vi "APD_filter.vi"(4 "error in":errorcluster, 5 "source of ticks":tag="/Dev1/100MHzTimebase", 6 "counter_filter":tag="Dev1/ctr1", 7 "APD signal":tag="/Dev1/PFI8") -> (0 "error out":errorcluster, 3 "filtered APD":refnum<k21>)   [LabVIEW 2018]
uses:
  <vilib>/DAQmx/create/channels.llb/DAQmx Create Channel (CO-Pulse Generation-Ticks).vi
  <vilib>/DAQmx/configure/trigger.llb/DAQmx Start Trigger (Digital Edge).vi
  <resource>/objmgr/daqmx.rc
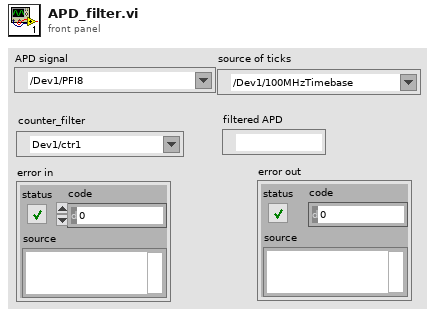
[diagram p1: front panel]
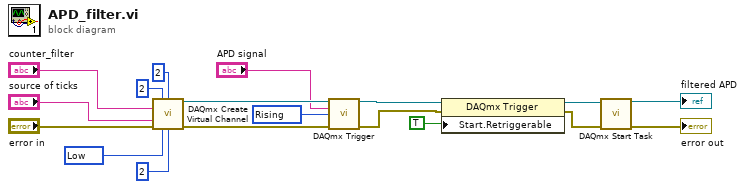
[diagram p0: block diagram]
diagram:
  w8 = 10280 items=["Rising"=10280, "Falling"=10171] ("edge")
  w6 = 10214 items=["High"=10192, "Low"=10214] ("idle state")
  n1 = call-poly <vilib>:"DAQmx Create Virtual Channel.vi"("high ticks"=u32 2, "low ticks"=u32 2, "counter"="counter_filter", "source of ticks"="source of ticks", "error in"="error in", "idle state"=w6, "initial delay"=u32 2) -> ("task out"=w12:refnum<k21>, "error out"=w15:errorcluster)  [unwired: 7 in]
  n2 = call-poly <vilib>:"DAQmx Trigger.vi"("task/channels in"=w12, "source"="APD signal", "edge"=w8, "error in"=w15) -> ("task out"=w10:refnum<k21>, "error out"=w16:errorcluster)  [unwired: 10 in]
  n3 = property class="DAQmx Trigger"(reference=w10, error in=w16, "Start.Retriggerable"=TRUE) -> (reference out=w13:refnum<k21>, error out=w17:errorcluster)
  n4 = call <vilib>:"DAQmx Start Task.vi"("task/channels in"=w13, "error in"=w17) -> ("task out"=→"filtered APD":refnum<k21>, "error out"=→"error out":errorcluster)  [unwired: 12 in]
